vi "add_bool.vi"   [LabVIEW 2014]
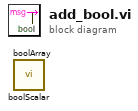
[diagram p0: block diagram]
diagram:
  n1 = call "boolScalar.vi"() -> ()  [unwired: 5 in, 1 out]
  n2 = call "boolArray.vi"() -> ()  [unwired: 5 in, 1 out]
